vi "Name to Item.vi"(8 "error in (no error)":errorcluster, 11 "itemName":string) -> (0 "error out":errorcluster, 3 ".NET Refnum out":refnum<k24>)   [LabVIEW 2024, in "LV_OPC_NET.lvlib"]
uses:
  C:/Users/Andrey/Desktop/LV_OPC-Client-x64/LV_OPC_Test/OPC.NET/OpcNetApi.dll
  OpcNetApi.dll
  LV_OPC_NET.lvlib
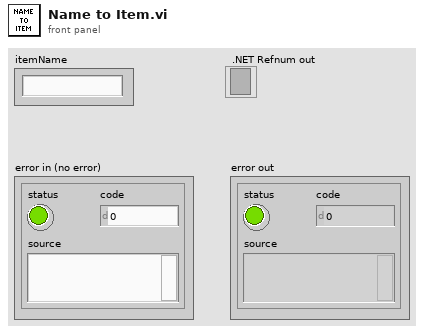
[diagram p1: front panel]
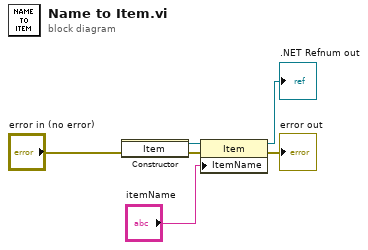
[diagram p0: block diagram]
diagram:
  n1 = constructor class="Item"(error in="error in (no error)") -> (reference out=w1:refnum<k24>, error out=w5:errorcluster)  [unwired: 2 in, 1 out]
  n2 = property class="Item"(reference=w1, error in=w5, "ItemName"="itemName") -> (reference out=→".NET Refnum out":refnum<k24>, error out=→"error out":errorcluster)
